vi "VG_OCV30min.vi"() -> ()   [LabVIEW 2020]
panel:
  out "OCV30min":dbl
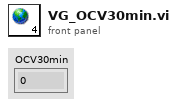
[diagram p1: front panel]
diagram:
